vi "scan2d_stepXY_coordinate.vi"(8 "error in (no error)":errorcluster, 10 "Step#":i32, 11 "scan_2d in":refnum<class "scan_2d.lvclass">) -> (0 "error out":errorcluster, 3 "scan_2d out":refnum<class "scan_2d.lvclass">)   [LabVIEW 2015, in "scan_2d.lvclass"]
uses:
  scan_2d.lvclass
  scan_2d.lvclass/scan_2d.ctl
  Stage Class/Stage.lvclass
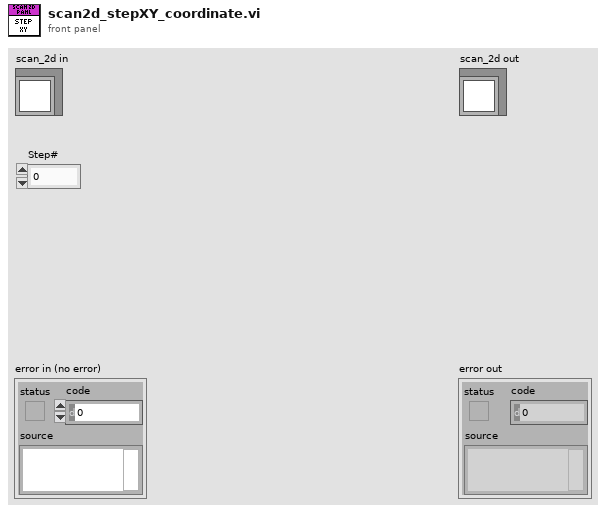
[diagram p1: front panel]
types:
  T1 = typedef "scan_coordinates_tdef.ctl" = cluster{"X":dbl, "Y":dbl, "Retrace?":bool}
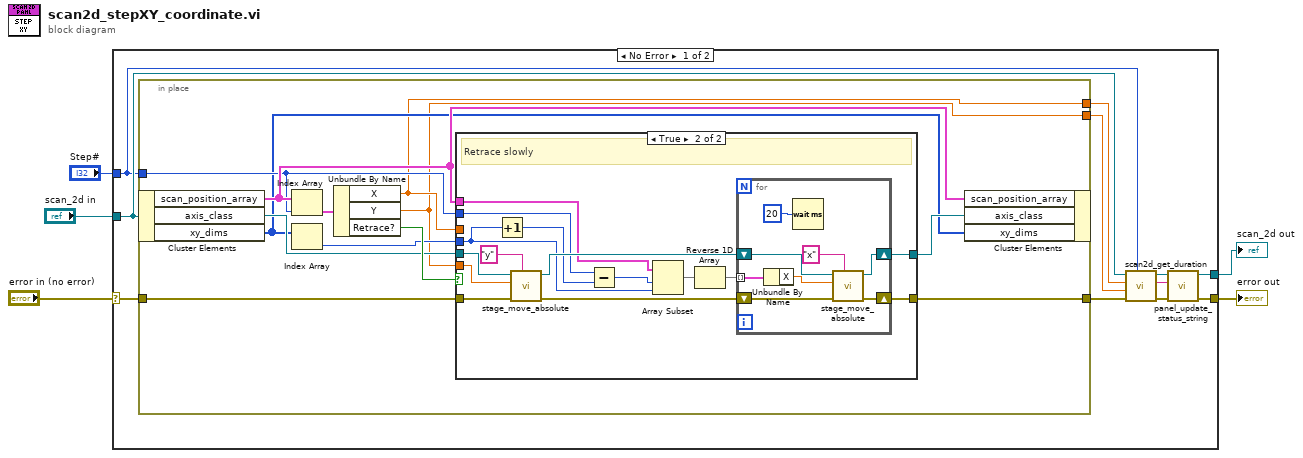
[diagram p0: block diagram]
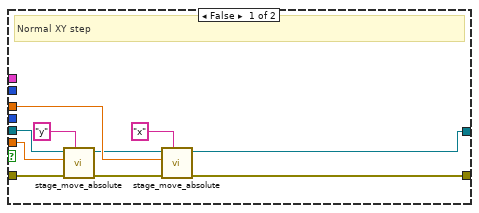
[diagram p2: hidden frame]
diagram:
  n1 = case shown="No Error" "error in (no error)" {
    selector: "error in (no error)" -> [w16 w63]
    tunnel: [w9 w63] -> w4
    tunnel: [w10 w62] -> w2
    tunnel: "scan_2d in" -> [w11 w62]
    tunnel: "Step#" -> [w6 _]
    frame No Error {
      n2 = in-place {
        in-place-border: w6 -> [w21]
        in-place-border: w16 -> [w26]
        in-place-border: [w23] -> w12
        in-place-border: [w18] -> w8
        in-place-border: [w17] -> w7
        n3 = in-place-cluster #1(w11) -> ("scan_position_array"=w22:T1[], "axis_class"=w25:refnum<class "Stage.lvclass">, "xy_dims"=w19:u32[])
        n4 = Index Array(array=w22, index=w21) -> (element=w27:T1)
        n5 = Index Array(array=w19) -> (element=w20:u32)  [unwired: 1 in]
        n6 = Unbundle By Name(w27) -> ("X"=w18:dbl, "Y"=w17:dbl, "Retrace?"=w28:bool)
        n7 = case shown="True" w28 {
          tunnel: w18 -> [w34 _]
          tunnel: w17 -> [w36 w47]
          tunnel: w26 -> [w37 w49]
          tunnel: [w31 w52] -> w23
          tunnel: [w30 w51] -> w24
          tunnel: w25 -> [w29 w39]
          tunnel: w22 -> [_ w42]
          tunnel: w21 -> [_ w41]
          tunnel: w20 -> [_ w40]
          frame False {
            # "Normal XY step"
            n8 = call-dynamic "stage_move_absolute.vi"("Stage Name"="y", "error in (no error)"=w37, "Position"=w36, "Stage in"=w29) -> ("error out"=w32:errorcluster, "Stage out"=w33:refnum<class "Stage.lvclass">)  [unwired: 6 in]
            n9 = call-dynamic "stage_move_absolute.vi"("Stage Name"="x", "error in (no error)"=w32, "Position"=w34, "Stage in"=w33) -> ("error out"=w31:errorcluster, "Stage out"=w30:refnum<class "Stage.lvclass">)  [unwired: 6 in]
          }
          frame True {
            # "Retrace slowly"
            n10 = Increment(x=w40) -> (x+1=w45:u32)
            n11 = call-dynamic "stage_move_absolute.vi"("Stage Name"="y", "error in (no error)"=w49, "Position"=w47, "Stage in"=w39) -> ("error out"=w48:errorcluster, "Stage out"=w46:refnum<class "Stage.lvclass">)  [unwired: 6 in]
            n12 = Subtract(x=w41, y=w45) -> (x-y=w53:u32)
            n13 = Array Subset(array=w42, index=w53, length=w40) -> (w44:T1[])
            n14 = Reverse 1D Array(array=w44) -> (reversed array=w43:T1[])
            n15 = for {
              tunnel: w43 -> [w55] mode=indexing
              shift-right: [w57] -> w51
              shift-left: w46 -> [w58]
              shift-right: [w59] -> w52
              shift-left: w48 -> [w60]
              n16 = Unbundle By Name(w55) -> ("X"=w54:dbl)
              n17 = Wait (ms)(milliseconds to wait=u32 20) -> ()  [unwired: 1 out]
              n18 = call-dynamic "stage_move_absolute.vi"("Stage Name"="x", "error in (no error)"=w60, "Position"=w54, "Stage in"=w58) -> ("error out"=w59:errorcluster, "Stage out"=w57:refnum<class "Stage.lvclass">)  [unwired: 6 in]
            }
          }
        }
        n19 = in-place-cluster #1("scan_position_array"=w22, "axis_class"=w24, "xy_dims"=w19) -> ()  [unwired: 1 out]
      }
      n20 = call "scan2d_get_duration.vi"("current_iteration"=w6, "error in (no error)"=w12, "current_y"=w7, "current_x"=w8, "scan_panel in"=w11) -> ("error out"=w15:errorcluster, "time_remaining"=w13:string, "scan_panel out"=w14:refnum<class "scan_2d.lvclass">)  [unwired: 4 in]
      n21 = call-dynamic "panel_update_status_string.vi"("error in (no error)"=w15, "String"=w13, "scan_panel in"=w14) -> ("error out"=w9:errorcluster, "scan_panel out"=w10:refnum<class "scan_2d.lvclass">)  [unwired: 7 in]
    }
    frame Error {
    }
  }
  "error out" <- w4
  "scan_2d out" <- w2
